vi "Open_HDF5 2D.vi"(0 "filename":path, 1 "log2 family size":i32=32, 2 "Compress":bool, 3 "sampling info":T1={"sample rate"=32000.0, "actual sample rate"=32000.0, "frame size"=8192.0} {"frame size" format="%.2f"; "sample rate" format="%.2f"}, 5 "channel names":string[](array[string]), 7 "gain":dbl=1000.0 format="%.2f", 9 "driver":u16(ring) items=["sec2", "stdio", "split", "family"], 11 "error in":errorcluster, 12 "chunk length":u32=16000, 13 "level":i32=9, 14 "cache specs":T3={"raw data cache size"=1000000, "raw data cache elements"=2000, "meta data cache elements"=5000, "w0"=0.75}) -> (4 "output cluster":T2, 15 "error out":errorcluster)   [LabVIEW 2010, in "HDF5.lvlib"]
uses:
  HDF5.lvlib
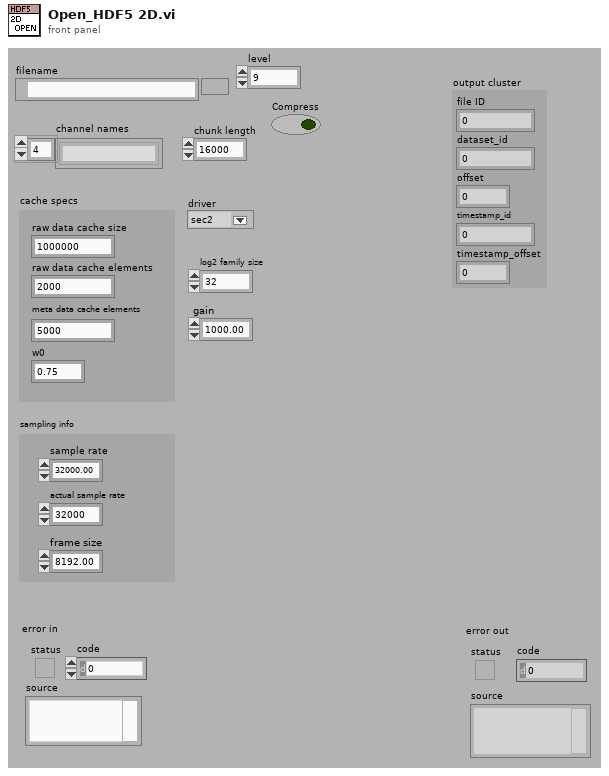
[diagram p1: front panel]
types:
  T1 = cluster{"sample rate":dbl, "actual sample rate":dbl, "frame size":dbl}
  T2 = cluster{"file ID":i32, "dataset_id":i32, "offset":dbl, "timestamp_id":i32, "timestamp_offset":dbl}
  T3 = cluster{"raw data cache size":u32, "raw data cache elements":i32, "meta data cache elements":i32, "w0":dbl}
  T4 = cluster{"file ID":i32, "dataset_id":i32, "offset":dbl, "dataset_id":i32, "offset":dbl}
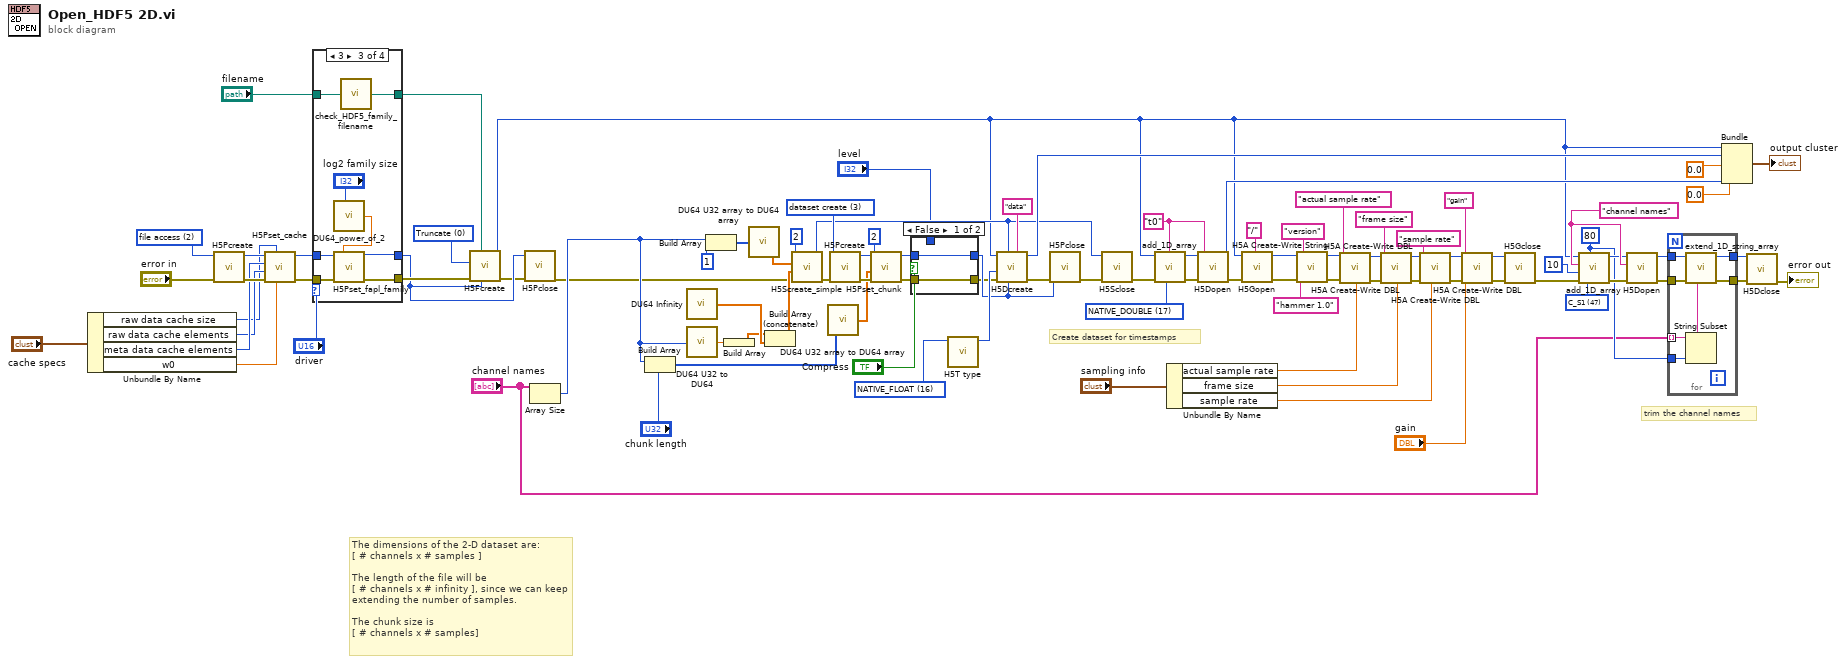
[diagram p0: block diagram]
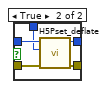
[diagram p2: hidden frame]
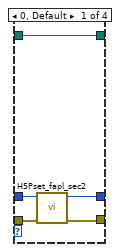
[diagram p3: hidden frame]
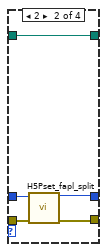
[diagram p4: hidden frame]
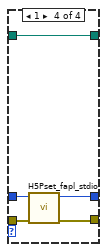
[diagram p5: hidden frame]
diagram:
  w32 = 17 items=["None", "IEEE_F32BE", "IEEE_F32LE", "IEEE_F64BE", "IEEE_F64LE", "NATIVE_CHAR", "NATIVE_SCHAR", "NATIVE_UCHAR", "NATIVE_SHORT", "NATIVE_USHORT", "NATIVE_INT", "NATIVE_UINT", "NATIVE_LONG", "NATIVE_ULONG", "NATIVE_LLONG", "NATIVE_ULLONG", "NATIVE_FLOAT", "NATIVE_DOUBLE", "NATIVE_LDOUBLE", "NATIVE_B8", "NATIVE_B16", "NATIVE_B32", "NATIVE_B64", "NATIVE_OPAQUE", "NATIVE_HADDR", "NATIVE_HSIZE", "NATIVE_HSSIZE", "NATIVE_HERR", "NATIVE_HBOOL", "STD_U8LE", "STD_U8BE", "STD_U16LE", "STD_U16BE", "STD_U32LE", "STD_U32BE", "STD_U64LE", "STD_U64BE", "STD_B8LE", "STD_B8BE", "STD_B16LE", "STD_B16BE", "STD_B32LE", "STD_B32BE", "STD_B64LE", "STD_B64BE", "STD_REF_OBJ", "STD_REF_DSETREG", "C_S1", "STD_I8LE", "STD_I8BE", "STD_I16LE", "STD_I16BE", "STD_I32LE", "STD_I32BE", "STD_I64LE", "STD_I64BE", ""] ("defined type")
  w51 = "channel names" ("dataset_name")
  w46 = u32 80 ("string length")
  w55 = 47 items=["None", "IEEE_F32BE", "IEEE_F32LE", "IEEE_F64BE", "IEEE_F64LE", "NATIVE_CHAR", "NATIVE_SCHAR", "NATIVE_UCHAR", "NATIVE_SHORT", "NATIVE_USHORT", "NATIVE_INT", "NATIVE_UINT", "NATIVE_LONG", "NATIVE_ULONG", "NATIVE_LLONG", "NATIVE_ULLONG", "NATIVE_FLOAT", "NATIVE_DOUBLE", "NATIVE_LDOUBLE", "NATIVE_B8", "NATIVE_B16", "NATIVE_B32", "NATIVE_B64", "NATIVE_OPAQUE", "NATIVE_HADDR", "NATIVE_HSIZE", "NATIVE_HSSIZE", "NATIVE_HERR", "NATIVE_HBOOL", "STD_U8LE", "STD_U8BE", "STD_U16LE", "STD_U16BE", "STD_U32LE", "STD_U32BE", "STD_U64LE", "STD_U64BE", "STD_B8LE", "STD_B8BE", "STD_B16LE", "STD_B16BE", "STD_B32LE", "STD_B32BE", "STD_B64LE", "STD_B64BE", "STD_REF_OBJ", "STD_REF_DSETREG", "C_S1", "STD_I8LE", "STD_I8BE", "STD_I16LE", "STD_I16BE", "STD_I32LE", "STD_I32BE", "STD_I64LE", "STD_I64BE", ""] ("defined type")
  w34 = "t0" ("name")
  w73 = 2 items=["no class", "file create", "file access", "dataset create", "dataset transfer", "mount", "n classes"] ("pclass")
  w86 = 16 items=["None", "IEEE_F32BE", "IEEE_F32LE", "IEEE_F64BE", "IEEE_F64LE", "NATIVE_CHAR", "NATIVE_SCHAR", "NATIVE_UCHAR", "NATIVE_SHORT", "NATIVE_USHORT", "NATIVE_INT", "NATIVE_UINT", "NATIVE_LONG", "NATIVE_ULONG", "NATIVE_LLONG", "NATIVE_ULLONG", "NATIVE_FLOAT", "NATIVE_DOUBLE", "NATIVE_LDOUBLE", "NATIVE_B8", "NATIVE_B16", "NATIVE_B32", "NATIVE_B64", "NATIVE_OPAQUE", "NATIVE_HADDR", "NATIVE_HSIZE", "NATIVE_HSSIZE", "NATIVE_HERR", "NATIVE_HBOOL", "STD_U8LE", "STD_U8BE", "STD_U16LE", "STD_U16BE", "STD_U32LE", "STD_U32BE", "STD_U64LE", "STD_U64BE", "STD_B8LE", "STD_B8BE", "STD_B16LE", "STD_B16BE", "STD_B32LE", "STD_B32BE", "STD_B64LE", "STD_B64BE", "STD_REF_OBJ", "STD_REF_DSETREG", "C_S1", "STD_I8LE", "STD_I8BE", "STD_I16LE", "STD_I16BE", "STD_I32LE", "STD_I32BE", "STD_I64LE", "STD_I64BE", ""] ("defined type")
  w87 = 3 items=["no class", "file create", "file access", "dataset create", "dataset transfer", "mount", "n classes"] ("pclass")
  w97 = 0 items=["Truncate", "Fail"] ("file access type")
  # "trim the channel names"
  # "Create dataset for timestamps"
  # "The dimensions of the 2-D dataset are:\n[ # channels x # samples ]\n\nThe length of the file will be\n[ # channels x # infinity ], since we can keep \nextending the number of samples.\n\nThe chunk size is \n[ # channels x # samples]"
  n1 = Unbundle By Name("cache specs") -> ("raw data cache size"=w21:u32, "raw data cache elements"=w22:i32, "meta data cache elements"=w23:i32, "w0"=w24:dbl)
  n2 = call "H5Pcreate.vi"("error in (no error)"="error in", "pclass"=w73) -> ("error out"=w72:errorcluster, "plist"=w74:i32)  [unwired: 8 out]
  n3 = call "H5Pset_cache.vi"("rdcc_w0"=w24, "rdcc_nbytes"=w21, "error in (no error)"=w72, "rdcc_elmts"=w22, "mdc_elmts"=w23, "plist in"=w74) -> ("error out"=w19:errorcluster, "plist out"=w17:i32)  [unwired: 4 in]
  n4 = case shown="3" "driver" {
    tunnel: w19 -> [w102 w105 w115 w118]
    tunnel: [w101 w107 w112 w117] -> w18
    tunnel: w17 -> [w100 w106 w114 w119]
    tunnel: [w99 w104 w113 w120] -> w16
    tunnel: [w98 w103 w108 w116] -> w13
    tunnel: "filename" -> [w98 w103 w109 w116]
    frame 0, Default {
      n5 = call "H5Pset_fapl_sec2.vi"("error in (no error)"=w102, "plist in"=w100) -> ("error out"=w101:errorcluster, "plist out"=w99:i32)  [unwired: 8 out]
    }
    frame 2 {
      n6 = call "H5Pset_fapl_split.vi"("plist in"=w106, "error in (no error)"=w105) -> ("plist out"=w104:i32, "error out"=w107:errorcluster)  [unwired: 4 in, 8 out]
    }
    frame 3 {
      n7 = call "DU64_power_of_2.vi"("x"="log2 family size") -> ("(DU64) 2^x"=w111:dbl)
      n8 = call "H5Pset_fapl_family.vi"("plist in"=w114, "memb_size"=w111, "error in (no error)"=w115) -> ("plist out"=w113:i32, "error out"=w112:errorcluster)  [unwired: 1 in, 10 out]
      n9 = call "check_HDF5_family_filename.vi"("Path"=w109) -> ("appended path"=w108:path)
    }
    frame 1 {
      n10 = call "H5Pset_fapl_stdio.vi"("error in (no error)"=w118, "plist in"=w119) -> ("error out"=w117:errorcluster, "plist out"=w120:i32)  [unwired: 8 out]
    }
  }
  n11 = call "H5Fcreate.vi"("access_id"=w16, "error in (no error)"=w18, "file access type"=w97, "filename"=w13) -> ("error out"=w15:errorcluster, "file ID"=w31:i32)  [unwired: 1 in, 5 out]
  n12 = call "H5Pclose.vi"("error in (no error)"=w15, "plist in"=w16) -> ("error out"=w66:errorcluster)  [unwired: 9 out]
  n13 = Array Size(array="channel names") -> (size(s)=w67:i32)
  n14 = Build Array(w67, "chunk length") -> (w81:u32[])
  n15 = call "DU64 Infinity.vi"() -> ("DU64 maxdims"=w77:dbl[])
  n16 = call "DU64 U32 to DU64.vi"("U32"=w67) -> ("DU64"=w79:dbl)
  n17 = Build Array(w67, u32 1) -> (w82:u32[])
  n18 = Build Array(w79) -> (w76:dbl[])
  n19 = call "DU64 U32 array to DU64 array.vi"("U32 array"=w82) -> ("DU64 array"=w92:dbl[])
  n20 = Build Array (concatenate)(w76, w77) -> (w90:dbl[])
  n21 = call "H5Screate_simple.vi"("error in (no error)"=w66, "DU64 maxdims"=w90, "DU64 dims"=w92, "rank"=2) -> ("error out"=w95:errorcluster, "space_id"=w39:i32)  [unwired: 6 out]
  n22 = call "DU64 U32 array to DU64 array.vi"("U32 array"=w81) -> ("DU64 array"=w91:dbl[])
  n23 = call "H5Pcreate.vi"("error in (no error)"=w95, "pclass"=w87) -> ("error out"=w94:errorcluster, "plist"=w96:i32)  [unwired: 8 out]
  n24 = call "H5Pset_chunk.vi"("error in (no error)"=w94, "DU64 dim"=w91, "ndims"=2, "plist in"=w96) -> ("error out"=w3:errorcluster, "plist out"=w6:i32)  [unwired: 6 out]
  n25 = case shown="False" "Compress" {
    tunnel: w6 -> [w122 w127]
    tunnel: [w122 w126] -> w5
    tunnel: [w121 w125] -> w4
    tunnel: w3 -> [w121 w124]
    tunnel: "level" -> [_ w123]
    frame False {
    }
    frame True {
      n26 = call "H5Pset_deflate.vi"("error in (no error)"=w124, "level"=w123, "plist in"=w127) -> ("error out"=w125:errorcluster, "plist out"=w126:i32)  [unwired: 7 out]
    }
  }
  n27 = call "H5T type.vi"("defined type"=w86) -> ("type_id"=w93:i32)  [unwired: 10 out]
  n28 = call "H5Dcreate.vi"("create_plist_id"=w5, "space_id"=w39, "error in (no error)"=w4, "type_id"=w93, "name"="data", "loc_id"=w31) -> ("error out"=w40:errorcluster, "dataset_id"=w84:i32)  [unwired: 4 out]
  n29 = call "H5Pclose.vi"("error in (no error)"=w40, "plist in"=w5) -> ("error out"=w85:errorcluster)  [unwired: 9 out]
  n30 = call "H5Sclose.vi"("error in (no error)"=w85, "space_id"=w39) -> ("error out"=w38:errorcluster)  [unwired: 9 out]
  n31 = call "add_1D_array.vi"("defined type"=w32, "error in (no error)"=w38, "dataset_name"=w34, "loc_id"=w31) -> ("error out"=w37:errorcluster, "dup loc_id"=w33:i32)  [unwired: 2 in, 4 out]
  n32 = Unbundle By Name("sampling info") -> ("actual sample rate"=w25:dbl, "frame size"=w43:dbl, "sample rate"=w42:dbl)
  n33 = call "H5Dopen.vi"("error in (no error)"=w37, "name"=w34, "loc_id"=w33) -> ("error out"=w36:errorcluster, "dataset_id"=w35:i32)  [unwired: 7 out]
  n34 = call "H5Gopen.vi"("error in (no error)"=w36, "name"="/", "loc_id"=w31) -> ("error out"=w63:errorcluster, "group_id"=w61:i32)  [unwired: 7 out]
  n35 = call "H5A Create-Write String.vi"("error in (no error)"=w63, "value"="hammer 1.0" ("String"), "attribute name"="version", "loc_id"=w61) -> ("error out"=w30:errorcluster, "dup loc_id"=w29:i32)  [unwired: 6 out]
  n36 = call "H5A Create-Write DBL.vi"("error in (no error)"=w30, "value"=w25, "attribute name"="actual sample rate", "loc_id"=w29) -> ("error out"=w27:errorcluster, "dup loc_id"=w28:i32)  [unwired: 6 out]
  n37 = call "H5A Create-Write DBL.vi"("error in (no error)"=w27, "value"=w43, "attribute name"="frame size", "loc_id"=w28) -> ("error out"=w58:errorcluster, "dup loc_id"=w59:i32)  [unwired: 6 out]
  n38 = call "H5A Create-Write DBL.vi"("error in (no error)"=w58, "value"=w42, "attribute name"="sample rate", "loc_id"=w59) -> ("error out"=w12:errorcluster, "dup loc_id"=w9:i32)  [unwired: 6 out]
  n39 = call "H5A Create-Write DBL.vi"("error in (no error)"=w12, "value"="gain", "attribute name"="gain", "loc_id"=w9) -> ("error out"=w11:errorcluster, "dup loc_id"=w10:i32)  [unwired: 6 out]
  n40 = call "H5Gclose.vi"("error in (no error)"=w11, "group_id"=w10) -> ("error out"=w56:errorcluster)  [unwired: 9 out]
  n41 = call "add_1D_array.vi"("defined type"=w55, "string length"=w46, "error in (no error)"=w56, "chunk size"=u32 10, "dataset_name"=w51, "loc_id"=w31) -> ("error out"=w53:errorcluster, "dup loc_id"=w50:i32)  [unwired: 4 out]
  n42 = call "H5Dopen.vi"("error in (no error)"=w53, "name"=w51, "loc_id"=w50) -> ("error out"=w52:errorcluster, "dataset_id"=w54:i32)  [unwired: 7 out]
  n43 = for {
    tunnel: w54 -> [w134]
    tunnel: w52 -> [w133]
    tunnel: [w132] -> w49
    tunnel: [w131] -> w47
    tunnel: w46 -> [w129]
    tunnel: "channel names" -> [w128] mode=indexing
    n44 = String Subset(string=w128, length (rest)=w129) -> (substring=w130:string)  [unwired: 1 out]
    n45 = call "extend_1D_string_array.vi"("String"=w130, "error in (no error)"=w133, "dataset_id"=w134) -> ("error out"=w132:errorcluster, "dup dataset_id"=w131:i32)  [unwired: 7 out]
  }
  n46 = Bundle("file ID"=w31, "dataset_id"=w84, "offset"=0.0, "dataset_id"=w35, "offset"=0.0) -> (→"output cluster":T4)  [unwired: 1 out]
  n47 = call "H5Dclose.vi"("error in (no error)"=w49, "dataset_id"=w47) -> ("error out"=→"error out":errorcluster)  [unwired: 9 out]
